vi "To AUT Stop.vi"(7 "Enqueuer ID":string, 8 "error in (no error)":errorcluster, 11 "Test Harness in":refnum<class "User Interface Tester.lvclass">) -> (0 "error out":errorcluster, 3 "Test Harness out":refnum<class "User Interface Tester.lvclass">)   [LabVIEW 2020, in "User Interface Tester.lvlib" / "User Interface Tester.lvclass"]
uses:
  User Interface Tester.lvclass
  User Interface Tester.lvclass/User Interface Tester.ctl
  <vilib>/ActorFramework/Message Enqueuer/Message Enqueuer.lvclass/Message Enqueuer.ctl
  <vilib>/ActorFramework/Message Enqueuer/Enqueue.vi
  <vilib>/ActorFramework/Stop Msg/Stop Msg.lvclass
  C:/Program Files (x86)/National Instruments/LabVIEW 2020/vi.lib/ActorFramework/Message/Message.lvclass
  <vilib>/ActorFramework/Message Priority Queue/Priority Enqueue.vi
  <vilib>/SAS/Actor Tester/Enqueuer Manager/SAS_AFTester_Enqueuer Manager.lvclass
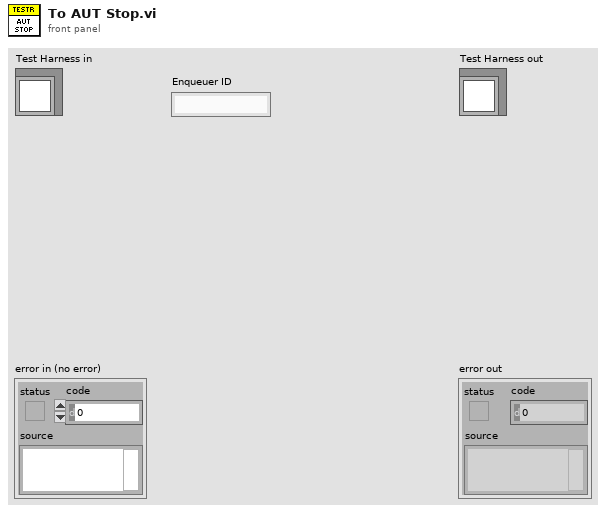
[diagram p1: front panel]
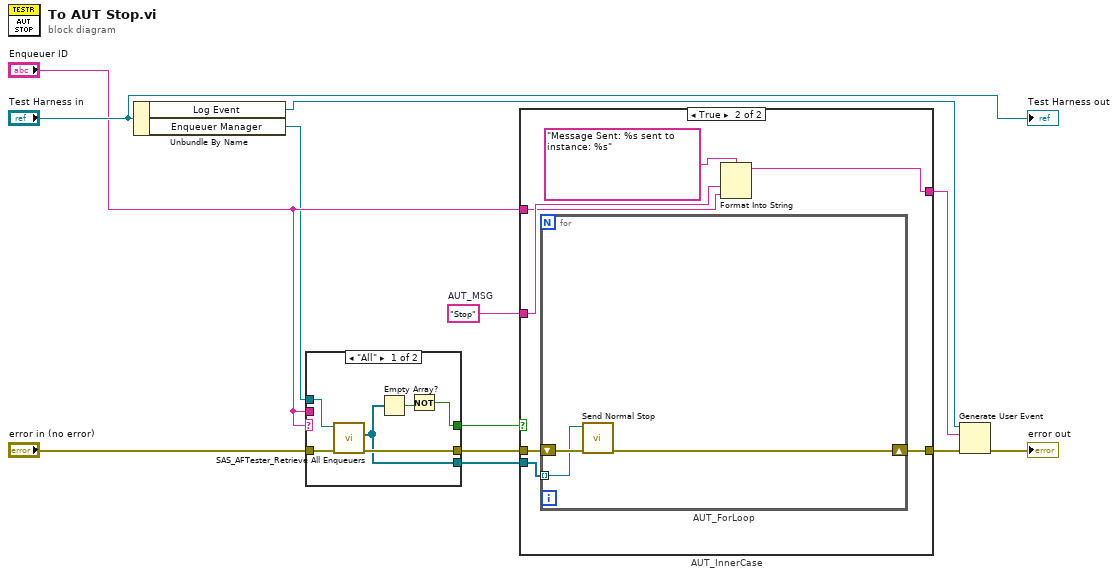
[diagram p0: block diagram]
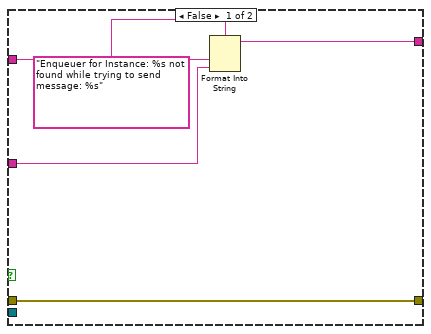
[diagram p2: hidden frame]
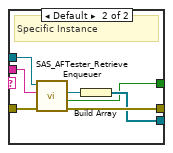
[diagram p3: hidden frame]
diagram:
  w2 = "Stop"  # AUT_MSG
  n1 = Unbundle By Name("Test Harness in") -> ("Log Event"=w4:refnum<user-event>, "Enqueuer Manager"=w8:refnum<class "SAS_AFTester_Enqueuer Manager.lvclass">)
  n2 = case shown="\"All\"" "Enqueuer ID" {
    tunnel: w8 -> [w18 w25]
    tunnel: "error in (no error)" -> [w17 w24]
    tunnel: [w16 w23] -> w7
    tunnel: "Enqueuer ID" -> [_ w22]
    tunnel: [w15 w20] -> w5
    tunnel: [w13 w19] -> w6
    frame "All" {
      n3 = call <vilib>:"SAS_AFTester_Retrieve All Enqueuers.vi"("error in (no error)"=w17, "Enqueuer Manager in"=w18) -> ("error out"=w16:errorcluster, "Enqueuers"=w15:refnum<class "Message Enqueuer.lvclass">[])  [unwired: 7 in, 1 out]
      n4 = Empty Array?(array=w15) -> (empty?=w14:bool)
      n5 = Not(x=w14) -> (.not. x?=w13:bool)
    }
    frame Default {
      # "Specific Instance"
      n6 = call <vilib>:"SAS_AFTester_Retrieve Enqueuer.vi"("error in (no error)"=w24, "Enqueuer ID"=w22, "Enqueuer Manager in"=w25) -> ("error out"=w23:errorcluster, "Found?"=w19:bool, "Message Enqueuer"=w21:refnum<class "Message Enqueuer.lvclass">)  [unwired: 5 in, 1 out]
      n7 = Build Array(w21) -> (w20:refnum<class "Message Enqueuer.lvclass">[])
    }
  }
  n8 = case "AUT_InnerCase" shown="True" w6 {
    tunnel: w7 -> [w30 w37]
    tunnel: w5 -> [_ w36]
    tunnel: [w30 w35] -> w3
    tunnel: w2 -> [w28 w32]
    tunnel: "Enqueuer ID" -> [w27 w31]
    tunnel: [w26 w33] -> w1
    frame False {
      n9 = Format Into String(format string="Enqueuer for Instance: %s not found while trying to send message: %s", w27, w28) -> (resulting string=w26:string)  [unwired: 2 in, 1 out]
    }
    frame True {
      n10 = for "AUT_ForLoop" {
        tunnel: w36 -> [w39] mode=indexing
        shift-right: [w38] -> w35
        shift-left: w37 -> [w40]
        n11 = call <vilib>:"Send Normal Stop.vi"("error in (no error)"=w40, "Message Enqueuer"=w39) -> ("error out"=w38:errorcluster)  [unwired: 9 in]
      }
      n12 = Format Into String(format string="Message Sent: %s sent to instance: %s", w32, w31) -> (resulting string=w33:string)  [unwired: 2 in, 1 out]
    }
  }
  n13 = Generate User Event(user event=w4, event data cluster=w1, error in=w3) -> (error out=→"error out":errorcluster)  [unwired: 1 in, 1 out]
  "Test Harness out" <- "Test Harness in"
